vi "LBCB Channels.vi"(9 "AreCommandChannels":bool, 11 "Task":refnum<k21>) -> ()   [LabVIEW 2013]
uses:
  <vilib>/Utility/miscctls.llb/LVRowAndColumnTypeDef.ctl
panel:
  in  "Ok":bool
  in  "LBCB Readings":string[](array[string])=["Stroke X1", "Stroke X2", "Stroke Y1", "Stroke Z1", "Stroke Z2", "Stroke Z3", "Load X1", "Load X2", "Load Y1", "Load Z1", "Load Z2", "Load Z3", "Servo X1", "Servo X2", "Servo Y1", "Servo Z1", "Servo Z2", "Servo Z3"]
  in  "LBCB Command Channels":string[](array[string])=["Command X1", "Command X2", "Command Y1", "Command Z1", "Command Z2", "Command Z3"]
  out "Task Name":string
  out "Channels":i32(listbox)
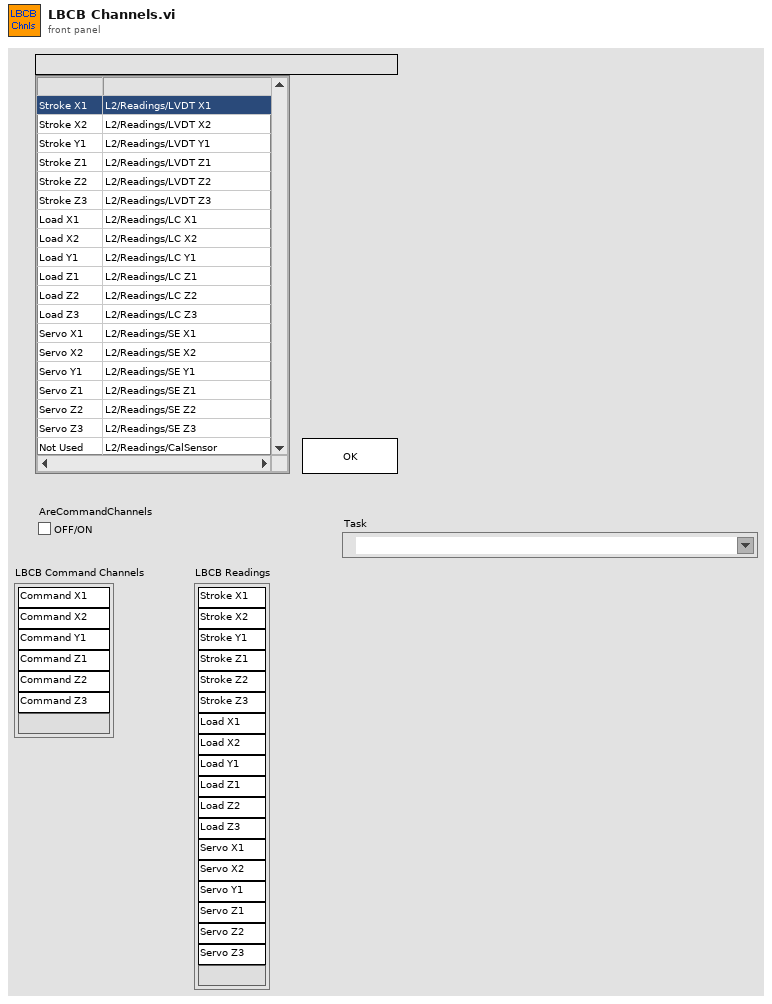
[diagram p1: front panel]
types:
  T1 = typedef "LVRowAndColumnTypeDef.ctl" = cluster{"Row":i32, "Column":i32}
  T2 = typedef "Compare Results.ctl" = enum16{"Lower", "Same", "Higher"}
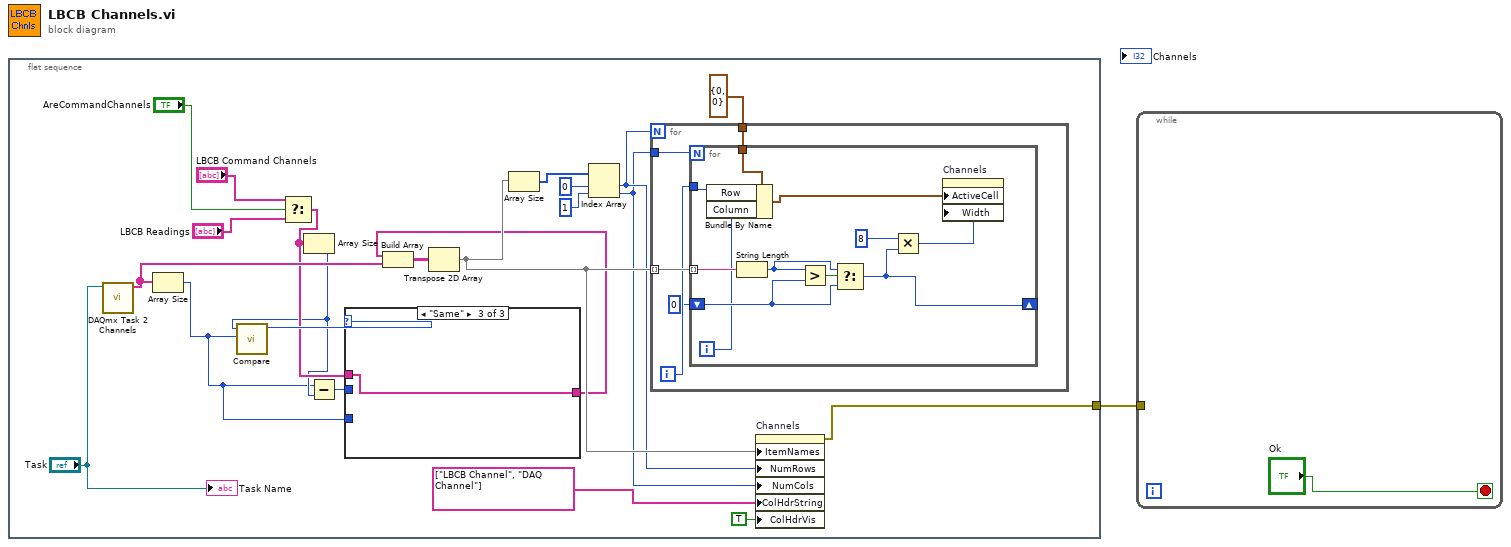
[diagram p0: block diagram]
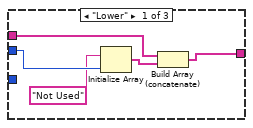
[diagram p2: hidden frame]
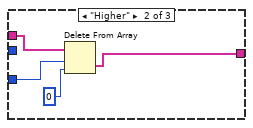
[diagram p3: hidden frame]
diagram:
  n1 = flat-sequence {
    tunnel: [w4] -> w1
    frame #0 {
      n2 = call "DAQmx Task 2 Channels.vi"("DAQmx Task Name"="Task") -> ("Channels Out"=w11:string[])  [unwired: 10 in]
      n3 = Array Size(array=w11) -> (size(s)=w5:i32)
      n4 = Select(t="LBCB Command Channels", s="AreCommandChannels", f="LBCB Readings") -> (s? t:f=w9:string[])
      n5 = Array Size(array=w9) -> (size(s)=w8:i32)
      n6 = call "Compare.vi"("Numeric 2"=w5, "Numeric 1"=w8) -> ("Result"=w10:T2)  [unwired: 9 in]
      n7 = Subtract(x=w5, y=w8) -> (x-y=w7:i32)
      n8 = case shown="\"Same\"" w10 {
        tunnel: w9 -> [w25 w32 w33]
        tunnel: w7 -> [w28 _ _]
        tunnel: [w24 w31 w33] -> w6
        tunnel: w5 -> [_ w30 _]
        frame "Lower" {
          n9 = Initialize Array("Not Used", w28) -> (w26:string[])
          n10 = Build Array (concatenate)(w25, w26) -> (w24:string[])
        }
        frame "Higher" {
          n11 = Delete From Array(array=w32, length=w30, index=0) -> (deleted portion=w31:string[])  [unwired: 1 out]
        }
        frame "Same" {
        }
      }
      n12 = Build Array(w6, w11) -> (w19:string[][])
      n13 = Transpose 2D Array(2D array=w19) -> (transposed array=w15:string[][])
      n14 = Array Size(array=w15) -> (size(s)=w18:i32[])
      n15 = Index Array(array=w18, index #1=0 ("index"), index #2=1 ("index")) -> (element #1=w13:i32, element #2=w12:i32)
      n16 = for {
        N: w13 -> [_]
        tunnel: w12 -> [w38]
        tunnel: w15 -> [w37] mode=indexing
        tunnel: T1 {"Row"=0, "Column"=0} ("Active Cell:Active Cell") -> [w36]
        i -> [w35]
        n17 = for {
          N: w38 -> [_]
          tunnel: w37 -> [w49] mode=indexing
          shift-right: [w41] -> _
          shift-left: 0 -> [w46]
          tunnel: w36 -> [w45]
          tunnel: w35 -> [w44]
          i -> [w43]
          n18 = Bundle By Name(cluster=w45, "Row"=w44, "Column"=w43) -> (w42:T1)
          n19 = String Length(string=w49) -> (length=w47:i32)
          n20 = Greater?(x=w47, y=w46) -> (0:w48:bool)
          n21 = Select(t=w47, s=w48, f=w46) -> (s? t:f=w41:i32)
          n22 = Multiply(x=8, y=w41) -> (x*y=w39:i32)
          n23 = property on="Channels" class="MCListbox (strict)"("ActiveCell"=w42, "Width"=w39) -> ()  [unwired: 2 in, 2 out]
        }
      }
      n24 = property on="Channels" class="MCListbox (strict)"("ItemNames"=w15, "NumRows"=w13, "NumCols"=w12, "ColHdrString"=string[] ["LBCB Channel", "DAQ Channel"] ("Column Header Strings[]"), "ColHdrVis"=TRUE ("Visible Items:Column Headers Visible")) -> (error out=w4:errorcluster)  [unwired: 2 in, 1 out]
      "Task Name" <- "Task"
    }
  }
  n25 = while {
    tunnel: w1 -> [_]
    stop <- "Ok" stop-if-true
  }
